vi "Error Memory Core.vi"(6 "Error Memory Core Enum":T1, 8 "error in (no error)":errorcluster, 11 "Error Code in":i32) -> (0 "error out":errorcluster, 1 "All Error Messages out":string[](array[string]), 2 "All Error Codes out":i32[](array[numeric]), 3 "Error Message out":string, 4 "All Errors Criticality out":u8[](array[numeric]), 5 "Error Criticality":u8)   [LabVIEW 2026, in "TALOS.lvlib" / "Error Memory.lvlib"]
doc: "This VI loads, at startup, all the custom errors in memory (TALOS_Error.xlsx only if not in PPL, TALOS_Error.xlsx and AEgIS_Errors.xlsx if inside the PPL). Then it can be called or to know the error message, given the error code, or to get the entire arrays of codes and messages, to create the pop-up using the General Error Handler."
uses:
  Error Memory.lvlib
  Error Memory Core Enum.ctl
  40c8088d-b597-4017-91af-faa98e00292e.vi
  d4a3ab98-063c-4e44-b43d-fbdcfe6c2be2.vi
  Support VIs/Global Memory.vi
  Support VIs/Global Constants.vi
  <vilib>/Comparison/Equal/Equal Functor/Equal Functor.lvclass
  TALOS.lvlib
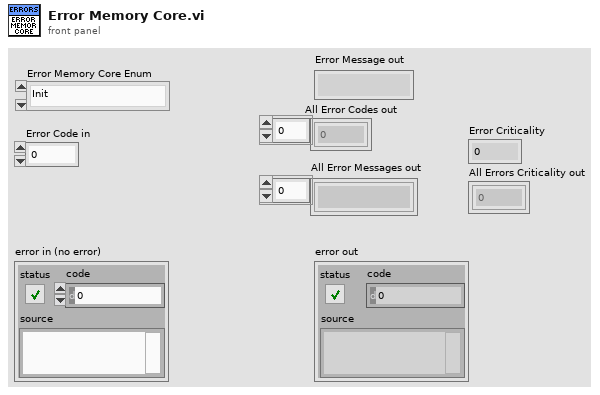
[diagram p1: front panel]
types:
  T1 = typedef "TALOS.lvlib/Error Memory.lvlib/Error Memory Core Enum.ctl" = enum16{"Init", "Get Error Message from Code", "Get All Errors", "Get Error Criticality from Code"}
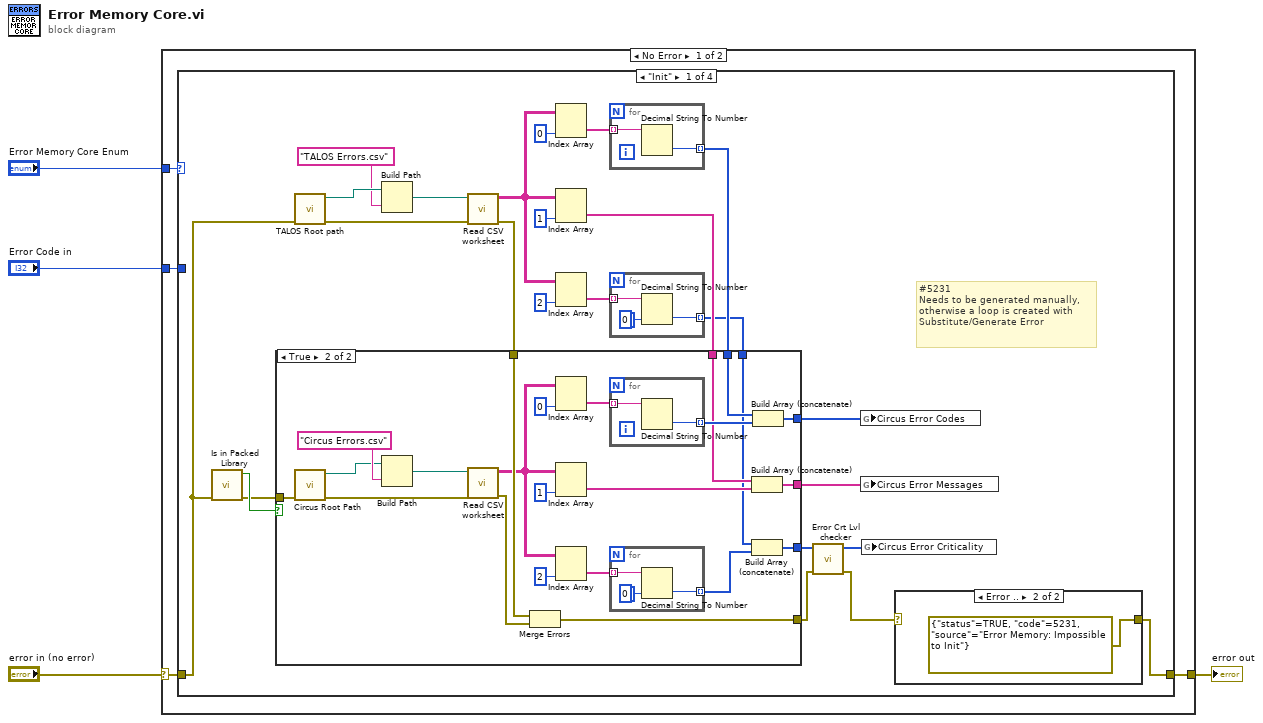
[diagram p0: block diagram]
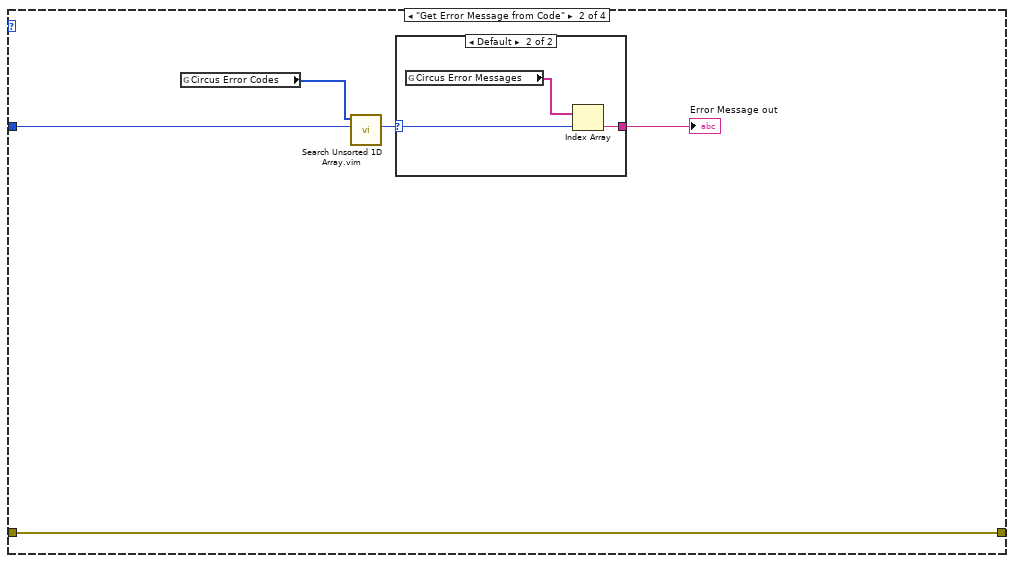
[diagram p4: hidden frame]
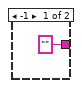
[diagram p5: hidden frame]
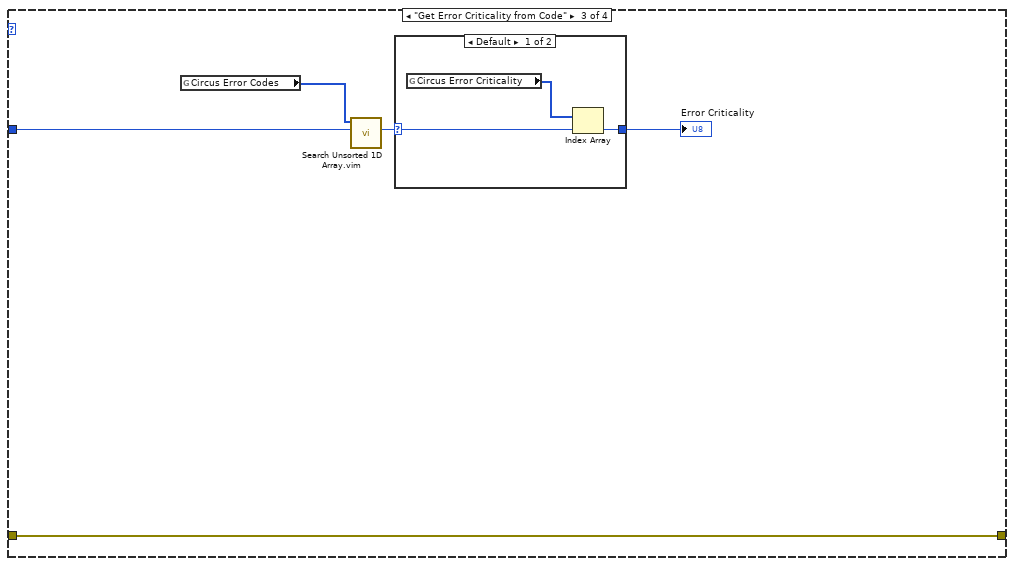
[diagram p6: hidden frame]
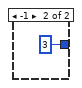
[diagram p7: hidden frame]
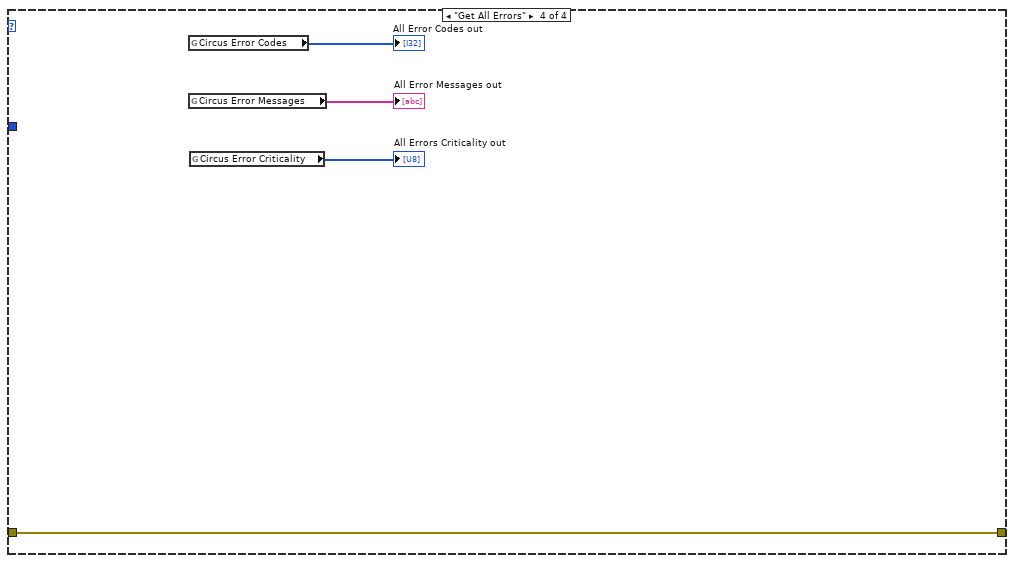
[diagram p8: hidden frame]
diagram:
  n1 = case shown="No Error" "error in (no error)" {
    selector: "error in (no error)" -> [w7 w94]
    tunnel: "Error Memory Core Enum" -> [w8 _]
    tunnel: [w6 w94] -> w2
    tunnel: "Error Code in" -> [w5 _]
    frame No Error {
      n2 = case shown="\"Init\"" w8 {
        tunnel: w7 -> [w18 w74 w84 w93]
        tunnel: [w17 w74 w84 w93] -> w6
        tunnel: w5 -> [_ w72 w82 _]
        frame "Init" {
          # "#5231\nNeeds to be generated manually, otherwise a loop is created with Substitute/Generate Error"
          n3 = call "Is in Packed Library.vi"("error in (no error)"=w18) -> ("error out"=w19:errorcluster, "Is In Packed Library"=w20:bool)  [unwired: 9 in]
          n4 = call "TALOS Root path.vi"("error in (no error)"=w18) -> ("error out"=w29:errorcluster, "TALOS Root Path"=w31:path)  [unwired: 9 in]
          n5 = Build Path(base path=w31, name or relative path="TALOS Errors.csv") -> (appended path=w32:path)
          n6 = call "Read CSV worksheet.vi"("error in (no error)"=w29, "appended path"=w32) -> ("error out"=w23:errorcluster, "Sheet"=w14:string[][])  [unwired: 8 in]
          n7 = Index Array(array=w14, index (col)=0 ("disabled index (col)")) -> (element=w26:string[])  [unwired: 1 in]
          n8 = Index Array(array=w14, index (col)=1 ("disabled index (col)")) -> (element=w24:string[])  [unwired: 1 in]
          n9 = Index Array(array=w14, index (col)=2 ("disabled index (col)")) -> (element=w15:string[])  [unwired: 1 in]
          n10 = for {
            tunnel: w26 -> [w37] mode=indexing
            tunnel: [w36] -> w25 mode=indexing
            n11 = Decimal String To Number(string=w37) -> (number=w36:i32)  [unwired: 2 in, 1 out]
          }
          n12 = for {
            tunnel: w15 -> [w35] mode=indexing
            tunnel: [w34] -> w13 mode=indexing
            n13 = Decimal String To Number(string=w35, default (0L)=u8 0 ("default (0 I32)")) -> (number=w34:u8)  [unwired: 1 in, 1 out]
          }
          n14 = case shown="True" w20 {
            tunnel: w19 -> [_ w64]
            tunnel: [w41 w52] -> w21
            tunnel: [w40 w51] -> w22
            tunnel: w25 -> [w41 w56]
            tunnel: w24 -> [w40 w54]
            tunnel: w23 -> [w39 w50]
            tunnel: [w39 w48] -> w10
            tunnel: w13 -> [w38 w45]
            tunnel: [w38 w42] -> w12
            frame False {
            }
            frame True {
              n15 = call "Circus Root Path.vi"("error in (no error)"=w64) -> ("error out"=w60:errorcluster, "Circus Root Path"=w62:path)  [unwired: 9 in]
              n16 = Build Path(base path=w62, name or relative path="Circus Errors.csv") -> (appended path=w61:path)
              n17 = call "Read CSV worksheet.vi"("error in (no error)"=w60, "appended path"=w61) -> ("error out"=w49:errorcluster, "Sheet"=w46:string[][])  [unwired: 8 in]
              n18 = Merge Errors(w50, w49) -> (w48:errorcluster)
              n19 = Index Array(array=w46, index (col)=0 ("disabled index (col)")) -> (element=w59:string[])  [unwired: 1 in]
              n20 = Index Array(array=w46, index (col)=1 ("disabled index (col)")) -> (element=w53:string[])  [unwired: 1 in]
              n21 = Index Array(array=w46, index (col)=2 ("disabled index (col)")) -> (element=w44:string[])  [unwired: 1 in]
              n22 = for {
                tunnel: w59 -> [w69] mode=indexing
                tunnel: [w68] -> w55 mode=indexing
                n23 = Decimal String To Number(string=w69) -> (number=w68:i32)  [unwired: 2 in, 1 out]
              }
              n24 = for {
                tunnel: w44 -> [w67] mode=indexing
                tunnel: [w66] -> w43 mode=indexing
                n25 = Decimal String To Number(string=w67, default (0L)=u8 0 ("default (0 I32)")) -> (number=w66:u8)  [unwired: 1 in, 1 out]
              }
              n26 = Build Array (concatenate)(w54, w53) -> (w51:string[])
              n27 = Build Array (concatenate)(w45, w43) -> (w42:u8[])
              n28 = Build Array (concatenate)(w56, w55) -> (w52:i32[])
            }
          }
          n29 = call "Error Crt Lvl checker.vi"("error in (no error)"=w10, "Array of Error Crt in"=w12) -> ("error out"=w9:errorcluster, "Array of Error Crt out"=w11:u8[])  [unwired: 8 in]
          n30 = global write "Global Memory.vi" "Circus Error Codes"(w21) -> ()
          n31 = global write "Global Memory.vi" "Circus Error Messages"(w22) -> ()
          n32 = global write "Global Memory.vi" "Circus Error Criticality"(w11) -> ()
          n33 = case shown="Error .." w9 {
            selector: w9 -> [w70 _]
            tunnel: [w70 errorcluster {"status"=TRUE, "code"=5231, "source"="Error Memory: Impossible to Init"} ("error IO")] -> w17
            frame No Error {
            }
            frame Error {
            }
          }
        }
        frame "Get Error Message from Code" {
          n34 = global read "Global Memory.vi" "Circus Error Codes"() -> (w73:i32[])
          n35 = call "Search Unsorted 1D Array.vim"("element"=w72, "unsorted 1D array"=w73) -> ("index of element"=w76:i32)  [unwired: 9 in]
          n36 = case shown="Default" w76 {
            selector: w76 -> [_ w80]
            tunnel: ["" w79] -> w75
            frame -1 {
            }
            frame Default {
              n37 = global read "Global Memory.vi" "Circus Error Messages"() -> (w78:string[])
              n38 = Index Array(array=w78, index=w80) -> (element=w79:string)
            }
          }
          "Error Message out" <- w75
        }
        frame "Get Error Criticality from Code" {
          n39 = global read "Global Memory.vi" "Circus Error Codes"() -> (w83:i32[])
          n40 = call "Search Unsorted 1D Array.vim"("element"=w82, "unsorted 1D array"=w83) -> ("index of element"=w85:i32)  [unwired: 9 in]
          n41 = case shown="Default" w85 {
            selector: w85 -> [w88 _]
            tunnel: [w86 u8 3] -> w81
            frame Default {
              n42 = global read "Global Memory.vi" "Circus Error Criticality"() -> (w87:u8[])
              n43 = Index Array(array=w87, index=w88) -> (element=w86:u8)
            }
            frame -1 {
            }
          }
          "Error Criticality" <- w81
        }
        frame "Get All Errors" {
          n44 = global read "Global Memory.vi" "Circus Error Codes"() -> (→"All Error Codes out":i32[])
          n45 = global read "Global Memory.vi" "Circus Error Messages"() -> (→"All Error Messages out":string[])
          n46 = global read "Global Memory.vi" "Circus Error Criticality"() -> (→"All Errors Criticality out":u8[])
        }
      }
    }
    frame Error {
    }
  }
  "error out" <- w2
